vi "Dashboard Loop.vi"(7 "connection ID":refnum<k16>) -> ()   [LabVIEW 2014]
uses:
  Common Code/Dashboard Display Data.ctl
  Common Code/AutonomousDBPacket.ctl
  Common Code/commandCluster.ctl
  Common Code/Roller Indicators.ctl
  Common Code/Roller Mode Enum.ctl
  Common Code/Auto Roller Commands.ctl
  Common Code/Inner Roller States.ctl
  Sensors/Pot Data.ctl
  Rollers/Untip Can States.ctl
  Common Code/Elevator Status.ctl
  Common Code/Elevator Mode.ctl
  Common Code/Auto Elevator Indicators.ctl
  Common Code/Elevator State.ctl
  Common Code/IMU Data.ctl
  navX-MXP Library/COMMON/TypeDefs/Value TypeDefs/navX NAVX_CAL_STATUS.ctl
  navX-MXP Library/COMMON/TypeDefs/Value TypeDefs/navX NAVX_OP_STATUS.ctl
  Common Code/Encoder Values SuperCluster.ctl
  Common Code/Encoder Values.ctl
  Common Code/Power and Diagnostic Data.ctl
  Common Code/Utilities/PDP Data.ctl
  Common Code/Utilities/PCM Data.ctl
  Common Code/Loop Timings.ctl
  Common Code/Ultrasonic Indicators.ctl
  Common Code/Drivetrain Status.ctl
  Drivetrain Code/Drivetrain Mode.ctl
  Common Code/Dist Drive Status.ctl
  Common Code/Yaw Rate Compensation Indicators.ctl
  Pike/Pike Indicators.ctl
  Pike/Pike State.ctl
  Pike/Pike Mode.ctl
  Elevator/Elevator Control Command.ctl
  Elevator/Elevator Command.ctl
  Common Code/Elevator Idle Mode.ctl
  Robot Global Data.vi
  navX-MXP Library/navX-MXP IMU.lvlib
panel:
  out "length":i32
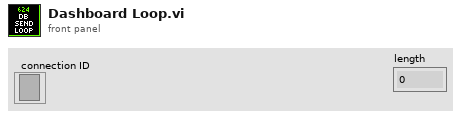
[diagram p1: front panel]
types:
  T1 = typedef "Loop Timings.ctl" = cluster{"Roller Loop":i32, "Elevator Loop":i32, "US Loop":i32, "100ms Loop":i32, "Drivetrain Loop":i32}
  T2 = typedef "Dashboard Display Data.ctl" = cluster{"Gyro Angle":dbl, "Autonomous":T3, "Pressure Transducer V":dbl, "Pressure":dbl, "Roller State Indicators":T5, "Elevator Status Data":T11, "IMU Data":T15, "Tote Count":i8, "Have Trashcan":bool, "Encoder Values":T18, "Power and Diagnostic Data":T20, "Loop Timings":T1, "Ultrasonic Data":T23, "Zeroing Rollers?":bool, "Drivetrain":T24, "Current Auto Command Data":T4, "Can Grabber":bool, "Pike":T28, "Elevator Command":T31}
  T3 = typedef "AutonomousDBPacket.ctl" = cluster{"Selected File":string, "Directory":string, "Auton File Index":i32, "Auton File Count":i32, "Auton Command Array":T4[]}
  T4 = typedef "commandCluster.ctl" = cluster{"Step ID":i16, "Command Type":i16, "Drive X":sgl, "Drive Y":sgl, "Heading":sgl, "Max Exec. Time":i16, "Jump Type":i32, "Jump To":i16, "Jump Condition":i16, "Async Drive?":i16, "Roller Mode":i16, "Roller Align":i16, "Roller Closed?":i16, "Wait Condition":i16, "Elevator Mode":i16, "Elevator Command":i16, "Roller State":i16, "Hold Low?":i16, "Num Totes":i16, "Num Cans":dbl, "Past Distance":dbl, "Store Can?":dbl, "X Speed":dbl, "Y Speed":dbl, "Yaw Angle Set":dbl, "Grab Can":dbl, "Roller Overide Speed":dbl, "Force Load?":sgl, "Set Idle":sgl, "Eject":sgl, "Pike Action":sgl, "Pivot Speed":dbl, "Height":dbl}
  T5 = typedef "Roller Indicators.ctl" = cluster{"Rollers Closed?":bool, "Roller Mode":T6, "Auto Roller State":T7, "Tote Inside?":bool, "Intake State":T8, "Left Ping Dist":sgl, "Right Ping Dist":sgl, "Potentiometer Cluster":T9, "PING Decision":T8, "Left Arm Closed?":bool, "Portrait?":bool, "Right Arm Closed?":bool, "Left Out":sgl, "Right Out":sgl, "Left Current":sgl, "Right Current":sgl, "Tote Load Complete?":bool, "Untip Complete?":bool, "Untip State":T10, "Roller Safety Open":bool}
  T6 = typedef "Roller Mode Enum.ctl" = enum16{"Manual", "Safe", "Auto"}
  T7 = typedef "Auto Roller Commands.ctl" = enum16{"Drag Tote", "Grab Tote", "Idle", "Eject Tote", "Untip Can", "Grab Can"}
  T8 = typedef "Inner Roller States.ctl" = enum16{"Turn Tote Portrait", "Acquire Tote", "Absorb Tote", "Turn Tote Right", "Turn Tote Left", "Acquire Can", "Absorb Can", "Turn Can", "Hold Tote"}
  T9 = typedef "Pot Data.ctl" = cluster{"Left Pot Zero":sgl, "Right Pot Zero":sgl, "Left Potentiometer":sgl, "Right Potentiometer":sgl, "Left Pot Non Zero":sgl, "Right Pot Non Zero":sgl}
  T10 = typedef "Untip Can States.ctl" = enum16{"Release Can", "Catch Can", "Idle"}
  T11 = typedef "Elevator Status.ctl" = cluster{"Height":dbl, "Enc Value":dbl, "Limit Override":bool, "Mode":T12, "High IR":bool, "Motor Out":dbl, "Ping Detect":bool, "Auto Elevator Indicators":T13, "Master Current":dbl, "Slave Current":dbl, "High Current":bool, "Current Tripped":bool, "Top Limit":bool, "Bottom Limit":bool, "Eject Piston":bool, "Stabilizer":bool, "Finger":bool, "Finger Height":dbl, "Finger Raw":dbl, "Finger at Bottom":bool}
  T12 = typedef "Elevator Mode.ctl" = enum16{"Manual", "Safe", "Auto"}
  T13 = typedef "Auto Elevator Indicators.ctl" = cluster{"Target Out":dbl, "Storing Trashcan?":bool, "State":T14, "In Range":bool, "Store Can Command":bool, "HP Load":bool}
  T14 = typedef "Elevator State.ctl" = enum16{"Idle", "Goto Load Position", "Wait for Load", "Load Drop", "Load Lift", "Drop Stack", "Goto Eject Position", "Eject ", "Raise Trashcan", "Open Stabilizer", "Untip Drop", "Untip Wait", "Untip Lift", "Abort Load", "HP Load Wait", "HP Load Drop", "HP Load Lift", "HP Load Abort", "Close Stabilizer", "HP Load Unfinish", "HP Load Score", "HP Load Finish", "HP Goto Finish Down", "HP Goto Finish Up"}
  T15 = typedef "IMU Data.ctl" = cluster{"Pitch":sgl, "Roll":sgl, "Yaw":sgl, "Data Valid?":bool, "Temp":sgl, "MOVING":bool, "NAVX_CAL_STATUS":T16, "NAVX_OP_STATUS":T17, "YAW_STABLE":bool, "Accel X":sgl, "Accel Y":sgl, "Accel Z":sgl, "Accel Magnitude":sgl, "Pitch Rate":sgl, "Roll Rate":sgl, "Yaw Rate":sgl, "NavX Opened?":bool}
  T16 = typedef "navX-MXP IMU.lvlib/navX NAVX_CAL_STATUS.ctl" = u8
  T17 = typedef "navX-MXP IMU.lvlib/navX NAVX_OP_STATUS.ctl" = u8
  T18 = typedef "Encoder Values SuperCluster.ctl" = cluster{"Left Encoder":T19, "Center Encoder":T19, "Right Encoder":T19}
  T19 = typedef "Encoder Values.ctl" = cluster{"Distance":dbl, "Speed":dbl, "Ticks":dbl}
  T20 = typedef "Power and Diagnostic Data.ctl" = cluster{"PDP Data":T21, "PCM Data":T22, "roboRIO input voltage (V)":dbl, "roboRIO input current (A)":dbl, "3.3V Rail Short":bool, "5 V Rail Short":bool, "6 V Rail Short":bool, "roboRIO Brownout":bool, "Outputs Enabled?":bool}
  T21 = typedef "PDP Data.ctl" = cluster{"Battery Voltage":sgl, "Temperature (degrees C)":sgl, "Internal Battery R (Ohms)":sgl, "Energy (J)":sgl, "Power (W)":sgl, "Total Current (A)":sgl, "Battery Voltage Fault":bool, "Temperature Fault":bool, "Hardware Fault":bool, "Currents":cluster{"[0]":sgl, "[1]":sgl, "[2]":sgl, "[3]":sgl, "[4]":sgl, "[5]":sgl, "[6]":sgl, "[7]":sgl, "[8]":sgl, "[9]":sgl, "[10]":sgl, "[11]":sgl, "[12]":sgl, "[13]":sgl, "[14]":sgl, "[15]":sgl}, "Current Faults":cluster{"[0]":bool, "[1]":bool, "[2]":bool, "[3]":bool, "[4]":bool, "[5]":bool, "[6]":bool, "[7]":bool, "[8]":bool, "[9]":bool, "[10]":bool, "[11]":bool, "[12]":bool, "[13]":bool, "[14]":bool, "[15]":bool}}
  T22 = typedef "PCM Data.ctl" = cluster{"Compressor Fault":bool, "Solenoid Fault":bool, "Compressor Enabled":bool, "Hardware Fault":bool, "Compressor Current":dbl}
  T23 = typedef "Ultrasonic Indicators.ctl" = cluster{"Left Distance":dbl, "Right Distance":dbl, "Center Distance":dbl, "Left Distance Unfilter":dbl, "Right Distance Unfilter":dbl, "Center Distance Unfilter":dbl}
  T24 = typedef "Drivetrain Status.ctl" = cluster{"Y (Throttle)":sgl, "X (Steer)":sgl, "Translation X":sgl, "Center Wheel Down":bool, "Mode":T25, "Distance Drive finished?":bool, "Y Target":sgl, "X Target":sgl, "Heading Target":sgl, "Dist Drive Status":T26, "Step Eject Lockout":bool, "Gyro In Range?":bool, "Yaw Comp Indicators":T27}
  T25 = typedef "Drivetrain Mode.ctl" = enum16{"Manual", "Gyro Steer", "Vision Steer", "Drive Distance", "Yaw Rate Compensate"}
  T26 = typedef "Dist Drive Status.ctl" = cluster{"Y In Range":bool, "X In Range":bool, "Gyro In Range":bool, "Y Dist":dbl, "X Dist":dbl, "Gyro":dbl}
  T27 = typedef "Yaw Rate Compensation Indicators.ctl" = cluster{"Rate Command":sgl, "Rate Actual":sgl, "Steer adjustment":sgl}
  T28 = typedef "Pike Indicators.ctl" = cluster{"Motor Out":dbl, "Current":dbl, "Limit Switch":bool, "Current Limit":bool, "State":T29, "Command":T30}
  T29 = typedef "Pike State.ctl" = enum16{"Up", "Down", "Going Up", "Going Down"}
  T30 = typedef "Pike Mode.ctl" = enum16{"Idle", "Auto Down", "Auto Up", "Manual Down", "Manual Up"}
  T31 = typedef "Elevator Control Command.ctl" = cluster{"Command":T32, "Manual Motor Out":dbl, "Manual Eject Piston":bool, "Mode":T12, "Override Limits":bool, "Manual Stabilizer":bool, "Manual Finger":bool, "Store Trashcan?":bool, "Hold Low?":bool, "Idle Mode":T33, "HP Load":bool, "Unstick":bool, "Raw Height Set":dbl}
  T32 = typedef "Elevator Command.ctl" = enum16{"Idle", "Load 1", "Load 2", "Load 3", "Drop Stack", "Eject Stack", "Untip Trashcan", "Load Trashcan", "HP Load", "HP Score"}
  T33 = typedef "Elevator Idle Mode.ctl" = enum16{"Load 1", "Load 2", "Load 3", "Load Can", "Untip Can", "Step Load", "Drop Stack", "Raw Height"}
  T34 = cluster{"Left Encoder":T19, "Center Encoder":T19, "Right Encoder":T19}
  T35 = cluster{"Motor Out":dbl, "Current":dbl, "Limit Switch":bool, "Current Limit":bool, "State":T29, "Command":T30}
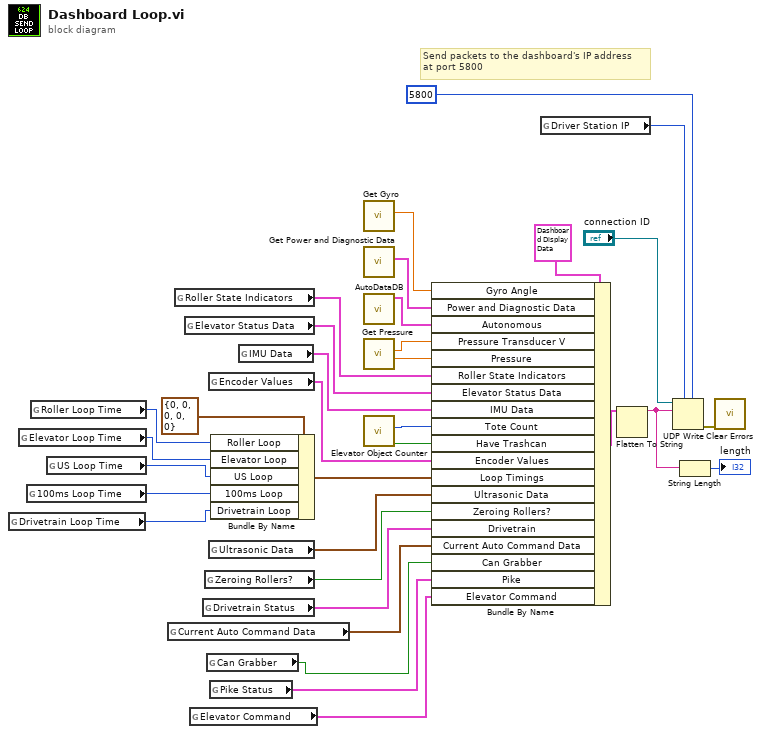
[diagram p0: block diagram]
diagram:
  # "Send packets to the dashboard's IP address\nat port 5800"
  n1 = global read "Robot Global Data.vi" "Drivetrain Loop Time"() -> (w7:i32)
  n2 = global read "Robot Global Data.vi" "Elevator Loop Time"() -> (w13:i32)
  n3 = global read "Robot Global Data.vi" "100ms Loop Time"() -> (w8:i32)
  n4 = global read "Robot Global Data.vi" "Roller Loop Time"() -> (w14:i32)
  n5 = global read "Robot Global Data.vi" "US Loop Time"() -> (w11:i32)
  n6 = global read "Robot Global Data.vi" "Current Auto Command Data"() -> (w6:T4)
  n7 = global read "Robot Global Data.vi" "Roller State Indicators"() -> (w26:T5)
  n8 = global read "Robot Global Data.vi" "Elevator Status Data"() -> (w22:T11)
  n9 = global read "Robot Global Data.vi" "Elevator Command"() -> (w1:T31)
  n10 = global read "Robot Global Data.vi" "Drivetrain Status"() -> (w9:T24)
  n11 = global read "Robot Global Data.vi" "Zeroing Rollers?"() -> (w10:bool)
  n12 = global read "Robot Global Data.vi" "Can Grabber"() -> (w3:bool)
  n13 = global read "Robot Global Data.vi" "Encoder Values"() -> (w18:T34)
  n14 = global read "Robot Global Data.vi" "Ultrasonic Data"() -> (w12:T23)
  n15 = global read "Robot Global Data.vi" "Pike Status"() -> (w2:T35)
  n16 = Bundle By Name(cluster=T1 {"Roller Loop"=0, "Elevator Loop"=0, "US Loop"=0, "100ms Loop"=0, "Drivetrain Loop"=0} ("Loop Timings"), "Roller Loop"=w14, "Elevator Loop"=w13, "US Loop"=w11, "100ms Loop"=w8, "Drivetrain Loop"=w7) -> (w15:T1)
  n17 = global read "Robot Global Data.vi" "IMU Data"() -> (w23:T15)
  n18 = call "Get Gyro.vi"() -> ("Angle"=w21:dbl)  [unwired: 11 in]
  n19 = call "Get Power and Diagnostic Data.vi"() -> ("Power and Diagnostic Data"=w17:T20)  [unwired: 11 in]
  n20 = call "AutoDataDB.vi"() -> ("output cluster"=w28:T3)  [unwired: 11 in]
  n21 = call "Get Pressure.vi"() -> ("Pressure"=w25:dbl, "Voltage"=w24:dbl)  [unwired: 10 in]
  n22 = call "Elevator Object Counter.vi"() -> ("Have Trashcan"=w19:bool, "Tote Count"=w20:i8)  [unwired: 10 in]
  n23 = Bundle By Name(cluster=T2 {"Gyro Angle"=0.0, "Autonomous"={"Selected File"="", "Directory"="", "Auton File Index"=0, "Auton File Count"=0, "Auton Command Array"=[]}, "Pressure Transducer V"=0.0, "Pressure"=0.0, "Roller State Indicators"={"Rollers Closed?"=FALSE, "Roller Mode"=enum."Manual", "Auto Roller State"=enum."Grab Tote", "Tote Inside?"=FALSE, "Intake State"=enum."Acquire Tote", "Left Ping Dist"=0.0, "Right Ping Dist"=0.0, "Potentiometer Cluster"={"Left Pot Zero"=0.0, "Right Pot Zero"=0.0, "Left Potentiometer"=0.0, "Right Potentiometer"=0.0, "Left Pot Non Zero"=0.0, "Right Pot Non Zero"=0.0}, "PING Decision"=enum."Acquire Tote", "Left Arm Closed?"=FALSE, "Portrait?"=FALSE, "Right Arm Closed?"=FALSE, "Left Out"=0.0, "Right Out"=0.0, "Left Current"=0.0, "Right Current"=0.0, "Tote Load Complete?"=FALSE, "Untip Complete?"=FALSE, "Untip State"=enum."Idle", "Roller Safety Open"=FALSE}, "Elevator Status Data"={"Height"=0.0, "Enc Value"=0.0, "Limit Override"=FALSE, "Mode"=enum."Manual", "High IR"=FALSE, "Motor Out"=0.0, "Ping Detect"=FALSE, "Auto Elevator Indicators"={"Target Out"=0.0, "Storing Trashcan?"=FALSE, "State"=enum."Idle", "In Range"=FALSE, "Store Can Command"=FALSE, "HP Load"=FALSE}, "Master Current"=0.0, "Slave Current"=0.0, "High Current"=FALSE, "Current Tripped"=FALSE, "Top Limit"=FALSE, "Bottom Limit"=FALSE, "Eject Piston"=FALSE, "Stabilizer"=FALSE, "Finger"=FALSE, "Finger Height"=0.0, "Finger Raw"=0.0, "Finger at Bottom"=FALSE}, "IMU Data"={"Pitch"=0.0, "Roll"=0.0, "Yaw"=0.0, "Data Valid?"=FALSE, "Temp"=0.0, "MOVING"=FALSE, "NAVX_CAL_STATUS"=0, "NAVX_OP_STATUS"=0, "YAW_STABLE"=FALSE, "Accel X"=0.0, "Accel Y"=0.0, "Accel Z"=0.0, "Accel Magnitude"=0.0, "Pitch Rate"=0.0, "Roll Rate"=0.0, "Yaw Rate"=0.0, "NavX Opened?"=FALSE}, "Tote Count"=0, "Have Trashcan"=FALSE, "Encoder Values"={"Left Encoder"={"Distance"=0.0, "Speed"=0.0, "Ticks"=0.0}, "Center Encoder"={"Distance"=0.0, "Speed"=0.0, "Ticks"=0.0}, "Right Encoder"={"Distance"=0.0, "Speed"=0.0, "Ticks"=0.0}}, "Power and Diagnostic Data"={"PDP Data"={"Battery Voltage"=0.0, "Temperature (degrees C)"=0.0, "Internal Battery R (Ohms)"=0.0, "Energy (J)"=0.0, "Power (W)"=0.0, "Total Current (A)"=0.0, "Battery Voltage Fault"=FALSE, "Temperature Fault"=FALSE, "Hardware Fault"=FALSE, "Currents"={"[0]"=0.0, "[1]"=0.0, "[2]"=0.0, "[3]"=0.0, "[4]"=0.0, "[5]"=0.0, "[6]"=0.0, "[7]"=0.0, "[8]"=0.0, "[9]"=0.0, "[10]"=0.0, "[11]"=0.0, "[12]"=0.0, "[13]"=0.0, "[14]"=0.0, "[15]"=0.0}, "Current Faults"={"[0]"=FALSE, "[1]"=FALSE, "[2]"=FALSE, "[3]"=FALSE, "[4]"=FALSE, "[5]"=FALSE, "[6]"=FALSE, "[7]"=FALSE, "[8]"=FALSE, "[9]"=FALSE, "[10]"=FALSE, "[11]"=FALSE, "[12]"=FALSE, "[13]"=FALSE, "[14]"=FALSE, "[15]"=FALSE}}, "PCM Data"={"Compressor Fault"=FALSE, "Solenoid Fault"=FALSE, "Compressor Enabled"=FALSE, "Hardware Fault"=FALSE, "Compressor Current"=0.0}, "roboRIO input voltage (V)"=0.0, "roboRIO input current (A)"=0.0, "3.3V Rail Short"=FALSE, "5 V Rail Short"=FALSE, "6 V Rail Short"=FALSE, "roboRIO Brownout"=FALSE, "Outputs Enabled?"=FALSE}, "Loop Timings"={"Roller Loop"=0, "Elevator Loop"=0, "US Loop"=0, "100ms Loop"=0, "Drivetrain Loop"=0}, "Ultrasonic Data"={"Left Distance"=0.0, "Right Distance"=0.0, "Center Distance"=0.0, "Left Distance Unfilter"=0.0, "Right Distance Unfilter"=0.0, "Center Distance Unfilter"=0.0}, "Zeroing Rollers?"=FALSE, "Drivetrain"={"Y (Throttle)"=0.0, "X (Steer)"=0.0, "Translation X"=0.0, "Center Wheel Down"=FALSE, "Mode"=enum."Manual", "Distance Drive finished?"=FALSE, "Y Target"=0.0, "X Target"=0.0, "Heading Target"=0.0, "Dist Drive Status"={"Y In Range"=FALSE, "X In Range"=FALSE, "Gyro In Range"=FALSE, "Y Dist"=0.0, "X Dist"=0.0, "Gyro"=0.0}, "Step Eject Lockout"=FALSE, "Gyro In Range?"=FALSE, "Yaw Comp Indicators"={"Rate Command"=0.0, "Rate Actual"=0.0, "Steer adjustment"=0.0}}, "Current Auto Command Data"={"Step ID"=0, "Command Type"=0, "Drive X"=0.0, "Drive Y"=0.0, "Heading"=0.0, "Max Exec. Time"=0, "Jump Type"=0, "Jump To"=0, "Jump Condition"=0, "Async Drive?"=0, "Roller Mode"=0, "Roller Align"=0, "Roller Closed?"=0, "Wait Condition"=0, "Elevator Mode"=0, "Elevator Command"=0, "Roller State"=0, "Hold Low?"=0, "Num Totes"=0, "Num Cans"=0.0, "Past Distance"=0.0, "Store Can?"=0.0, "X Speed"=0.0, "Y Speed"=0.0, "Yaw Angle Set"=0.0, "Grab Can"=0.0, "Roller Overide Speed"=0.0, "Force Load?"=0.0, "Set Idle"=0.0, "Eject"=0.0, "Pike Action"=0.0, "Pivot Speed"=0.0, "Height"=0.0}, "Can Grabber"=FALSE, "Pike"={"Motor Out"=0.0, "Current"=0.0, "Limit Switch"=FALSE, "Current Limit"=FALSE, "State"=enum."Going Up", "Command"=enum."Auto Up"}, "Elevator Command"={"Command"=enum."Idle", "Manual Motor Out"=0.0, "Manual Eject Piston"=FALSE, "Mode"=enum."Manual", "Override Limits"=FALSE, "Manual Stabilizer"=FALSE, "Manual Finger"=FALSE, "Store Trashcan?"=FALSE, "Hold Low?"=FALSE, "Idle Mode"=enum."Load Can", "HP Load"=FALSE, "Unstick"=FALSE, "Raw Height Set"=0.0}} ("Cluster"), "Gyro Angle"=w21, "Power and Diagnostic Data"=w17, "Autonomous"=w28, "Pressure Transducer V"=w24, "Pressure"=w25, "Roller State Indicators"=w26, "Elevator Status Data"=w22, "IMU Data"=w23, "Tote Count"=w20, "Have Trashcan"=w19, "Encoder Values"=w18, "Loop Timings"=w15, "Ultrasonic Data"=w12, "Zeroing Rollers?"=w10, "Drivetrain"=w9, "Current Auto Command Data"=w6, "Can Grabber"=w3, "Pike"=w2, "Elevator Command"=w1) -> (w29:T2)
  n24 = global read "Robot Global Data.vi" "Driver Station IP"() -> (w33:u32)
  n25 = Flatten To String(anything=w29) -> (data string=w5:string)  [unwired: 3 in, 2 out]
  n26 = UDP Write(address=w33, port or service name=u16 5800, connection ID="connection ID", data in=w5) -> (error out=w32:errorcluster)  [unwired: 2 in, 1 out]
  n27 = String Length(string=w5) -> (length=→"length":i32)
  n28 = call <vilib>:"Clear Errors.vi"("error in (no error)"=w32) -> ()  [unwired: 5 in, 2 out]
